vi "YAFTAF_GetPersistentConfiguration.vi"(8 "ErrorIn":errorcluster, 10 "CmdData":variant, 11 "LocalIn":refnum<class>) -> (0 "ErrorOut":errorcluster, 2 "ReplyData":variant, 3 "LocalIn":refnum<class>, 4 "Exit":bool)   [LabVIEW 2021, in "YAFTAF.lvclass"]
uses:
  YAFTAF.lvclass
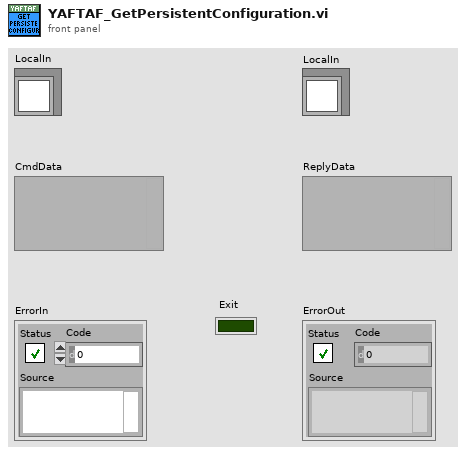
[diagram p1: front panel]
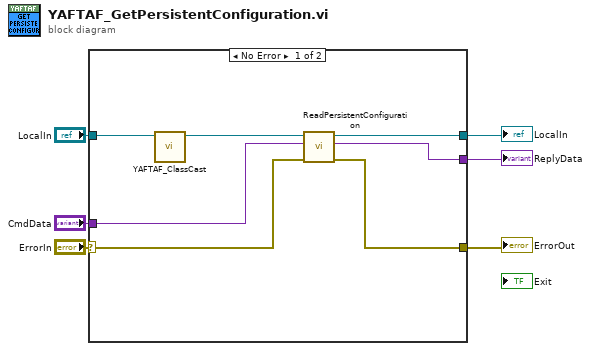
[diagram p0: block diagram]
diagram:
  n1 = case shown="No Error" "ErrorIn" {
    selector: "ErrorIn" -> [w12 w16]
    tunnel: [w13 w16] -> w5
    tunnel: [w9 w15] -> w3
    tunnel: "CmdData" -> [w7 w15]
    tunnel: "LocalIn" -> [w11 w14]
    tunnel: [w8 w14] -> w1
    frame No Error {
      n2 = call "YAFTAF_ClassCast.vi"("LocalIn"=w11) -> ("LocalOut"=w10:refnum<class "YAFTAF.lvclass">)  [unwired: 10 in]
      n3 = call-dynamic "ReadPersistentConfiguration.vi"("ErrorIn"=w12, "DataIn"=w7, "ObjectIn"=w10) -> ("ErrorOut"=w13:errorcluster, "DataOut"=w9:variant, "ObjectOut"=w8:refnum<class "YAFTAF.lvclass">)  [unwired: 6 in]
    }
    frame Error {
    }
  }
  "ErrorOut" <- w5
  "LocalIn" <- w1
  "ReplyData" <- w3
